vi "Save Data.vi"(8 "数据标记":string, 9 "测试人员":string, 10 "扫描数据":dbl[][](array[numeric]), 11 "时间标识":timestamp) -> (6 "保存失败":bool)   [LabVIEW 2020]
uses:
  <vilib>/Utility/error.llb/Error Cluster From Error Code.vi
  <vilib>/Utility/file.llb/Write Delimited Spreadsheet (DBL).vi
  <vilib>/ErrorRing/Error Ring.xnode
panel:
  # "文件名：日期-时间-数据标记"
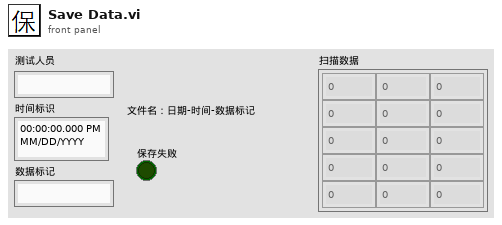
[diagram p1: front panel]
types:
  T1 = cluster{"status":bool, "code":bool, "source":bool}
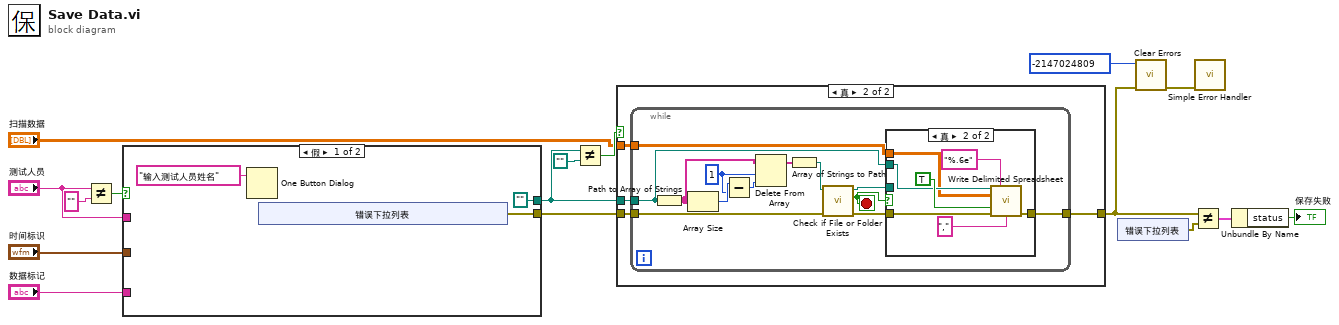
[diagram p0: block diagram]
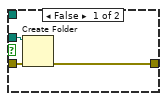
[diagram p3: hidden frame]
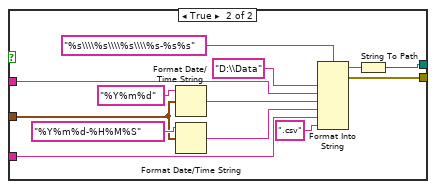
[diagram p4: hidden frame]
diagram:
  n1 = Not Equal?(x="测试人员", y="") -> (x != y?=w14:bool)
  n2 = case shown="假" w14 {
    tunnel: [path "" w33] -> w13
    tunnel: "测试人员" -> [_ w32]
    tunnel: "数据标记" -> [_ w28]
    tunnel: "时间标识" -> [_ w26]
    tunnel: [w17 w24] -> w7
    frame False {
      n3 = One Button Dialog(message="输入测试人员姓名" ("消息")) -> ()  [unwired: 1 in, 1 out]
      n4 = xnode "错误下拉列表"() -> ("错误输出"=w17:errorcluster)
    }
    frame True {
      n5 = Format Date/Time String(time format string (%c)="%Y%m%d" ("时间格式字符串(%c)"), seconds (now)=w26) -> (date/time string=w30:string)  [unwired: 1 in]
      n6 = Format Date/Time String(time format string (%c)="%Y%m%d-%H%M%S" ("时间格式字符串(%c)"), seconds (now)=w26) -> (date/time string=w29:string)  [unwired: 1 in]
      n7 = Format Into String(format string="%s\\\\%s\\\\%s\\\\%s-%s%s" ("格式字符串"), "D:\\Data", w32, w30, w29, w28, ".csv") -> (resulting string=w36:string, error out=w24:errorcluster)  [unwired: 2 in]
      n8 = String To Path(string=w36) -> (path=w33:path)
    }
  }
  n9 = Not Equal?(x=w13, y=path "") -> (x != y?=w11:bool)
  n10 = case shown="真" w11 {
    tunnel: w13 -> [_ w41]
    tunnel: "扫描数据" -> [_ w40]
    tunnel: [w37 w39] -> w3
    tunnel: w7 -> [w37 w38]
    frame False {
    }
    frame True {
      n11 = while {
        tunnel: w41 -> [w54]
        tunnel: w40 -> [w44]
        tunnel: [w43] -> w39
        tunnel: w38 -> [w42]
        stop <- w47 stop-if-true
        w51 = 1 ("长度")
        n12 = Path to Array of Strings(0:w54) -> (2:w53:string[])  [unwired: 1 out]
        n13 = Array Size(array=w53) -> (size(s)=w52:i32)
        n14 = Subtract(x=w52, y=w51) -> (x-y=w50:i32)
        n15 = Delete From Array(array=w53, length=w51, index=w50) -> (array with subset deleted=w49:string[])  [unwired: 1 out]
        n16 = Array of Strings to Path(0:w49) -> (2:w48:path)  [unwired: 1 in]
        n17 = call <vilib>:"Check if File or Folder Exists.vi"("error in (no error)"=w42, "path"=w48) -> ("error out"=w45:errorcluster, "file or folder exists?"=w47:bool, "dup path"=w46:path)  [unwired: 7 in]
        n18 = case shown="真" w47 {
          tunnel: w54 -> [_ w61]
          tunnel: w46 -> [w57 _]
          tunnel: w45 -> [w56 w59]
          tunnel: w44 -> [_ w60]
          tunnel: [w55 w58] -> w43
          frame False {
            n19 = Create Folder(path (use dialog)=w57, error in=w56) -> (error out=w55:errorcluster)  [unwired: 1 in, 2 out]
          }
          frame True {
            n20 = call-poly <vilib>:"Write Delimited Spreadsheet.vi"("file path (dialog if empty)"=w61, "format (%.3f)"="%.6e", "2D data"=w60, "append to file? (new file:F)"=TRUE, "error in (no error)"=w59, "delimiter (\\t)"="," ("delimiter (\\t)")) -> ("error out"=w58:errorcluster)  [unwired: 8 in, 1 out]
          }
        }
      }
    }
  }
  n21 = xnode "错误下拉列表"() -> ("错误输出"=w6:errorcluster)
  n22 = call <vilib>:"Clear Errors.vi"("error in (no error)"=w3, "specific error code to clear (0: all)"=-2147024809) -> ("error out"=w2:errorcluster)  [unwired: 4 in, 1 out]
  n23 = Not Equal?(x=w3, y=w6) -> (x != y?=w5:T1)
  n24 = call <vilib>:"Simple Error Handler.vi"("error in (no error)"=w2) -> ()  [unwired: 4 in, 5 out]
  n25 = Unbundle By Name(w5) -> ("status"=→"保存失败":bool)
